vi "Write readInitialTime.vi"(8 "error in (no error)":errorcluster, 10 "readInitialTime":dbl, 11 "State in":refnum<class "ElectrometerState.lvclass">) -> (0 "error out":errorcluster, 3 "State out":refnum<class "ElectrometerState.lvclass">)   [LabVIEW 2016, in "ElectrometerState.lvclass"]
uses:
  ElectrometerState.lvclass
  ElectrometerState.lvclass/ElectrometerState.ctl
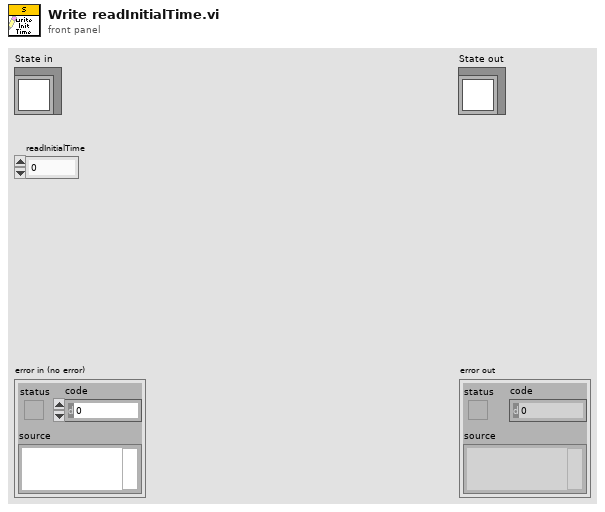
[diagram p1: front panel]
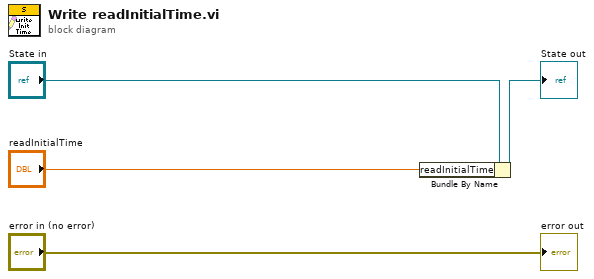
[diagram p0: block diagram]
diagram:
  n1 = Bundle By Name(cluster="State in", "readInitialTime"="readInitialTime") -> (→"State out":refnum<class "ElectrometerState.lvclass">)
  "error out" <- "error in (no error)"
